vi "BLED1112-Rx Packet parser (EVENT-Attribute Client).vi"(5 "message package":u8[](array[numeric])=[128, 13, 4, 5, 0, 18, 0, 1, 8, 32, 32, 51, 48, 49, 54, 13, 10] format="%02x") -> (0 "message out":u8[](array[numeric])=[128, 13, 4, 5, 0, 18, 0, 1, 8, 32, 32, 51, 48, 49, 54, 13, 10] format="%02x", 1 "Packet OK":bool, 2 "Data Structure":T1={"Message Type (Response)"=128, "Payload length"=16, "Command Class (System)"=3, "Message ID"=0, "Connection handle"=0, "Attribute handle"=50697, "Attribute type"=109, "Attribute value (data)"=[234, 23, 0, 0, 6, 0, 100, 0, 0, 0, 255]} {"Attribute type" format="%02x" items=["read", "notify", "indicate", "read_by_type", "read_blob", "indicate_rsp_req"]; "Attribute value (data)" format="%02x"; "Attribute handle" format="%04x"; "Connection handle" format="%02x"; "Message ID" format="%02x"; "Message Type (Response)" format="%02x" items=["Command / Response"=0, "Event"=128]; "Command Class (System)" format="%02x" items=["System", "Persistent Store", "Attribute database", "Connection", "Attribute client", "Security Manager", "Generic Access Profile", "Hardware"]})   [LabVIEW 2015]
uses:
  Control-BLED Rx (EVENT-Attribute Client).ctl
  Lib_Bled112 toolkit/type_def/message_type.ctl
  Lib_Bled112 toolkit/type_def/message_class.ctl
panel:
  # "Rx Packet parser (EVENT-Attribute Client)"
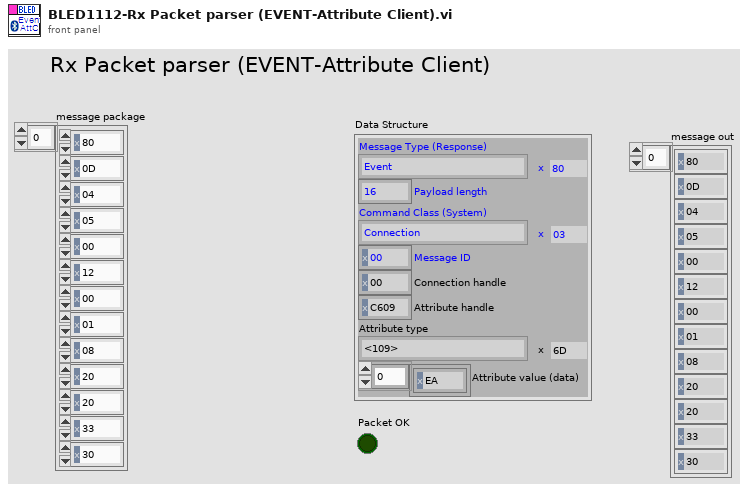
[diagram p1: front panel]
types:
  T1 = typedef "Control-BLED Rx (EVENT-Attribute Client).ctl" = cluster{"Message Type (Response)":T2, "Payload length":u8, "Command Class (System)":T3, "Message ID":u8, "Connection handle":u8, "Attribute handle":u16, "Attribute type":T3, "Attribute value (data)":u8[]}
  T2 = typedef "message_type.ctl" = u8
  T3 = typedef "message_class.ctl" = u8
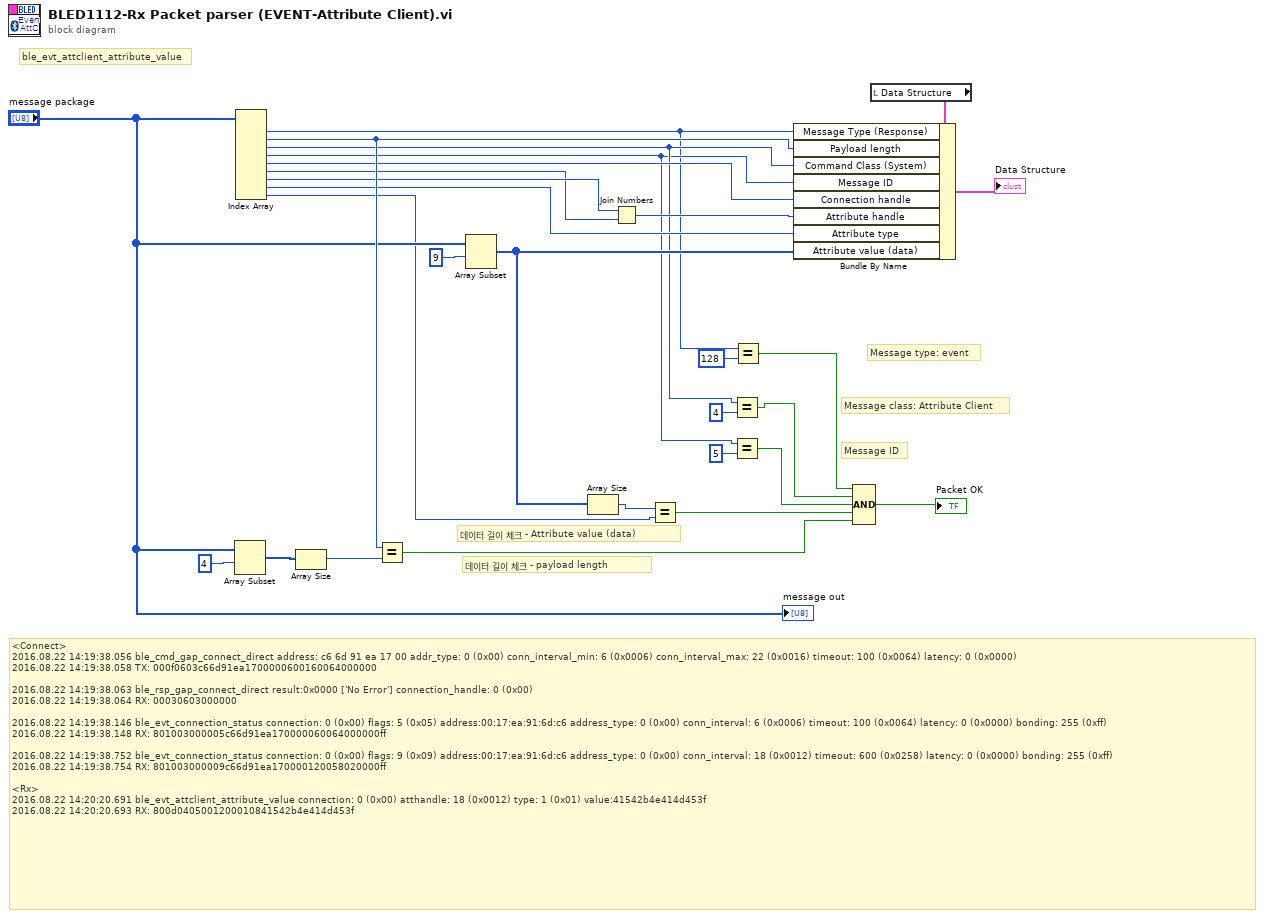
[diagram p0: block diagram]
diagram:
  # "Message type: event"
  # "Message ID"
  # "Message class: Attribute Client"
  # "데이터 길이 체크 - payload length"
  # "ble_evt_attclient_attribute_value"
  # "데이터 길이 체크 - Attribute value (data)"
  # "<Connect>\n2016.08.22 14:19:38.056 ble_cmd_gap_connect_direct address: c6 6d 91 ea 17 00 addr_type: 0 (0x00) conn_interval_min: 6 (0x0006) conn_interval_max: 22 (0x0016) timeout: 100 (0x0064) latency: 0 (0x0000)\n2016.08.22 14:19:38.058 TX: 000f0603c66d91ea1700000600160064000000\n\n2016.08.22 14:19:38.063 ble_rsp_gap_connect_direct result:0x0000 ['No Error'] connection_handle: 0 (0x00)\n2016.08.22 14:19:38.064 RX: 00030603000000\n\n2016.08.22 14:19:38.146 ble_evt_connection_status connection: 0 (0x00) flags: 5 (0x05) address:00:17:ea:91:6d:c6 address_type: 0 (0x00) conn_interval: 6 (0x0006) timeout: 100 (0x0064) latency: 0 (0x0000) bonding: 255 (0xff)\n2016.08.22 14:19:38.148 RX: 801003000005c66d91ea170000060064000000ff\n\n2016.08.22 14:19:38.752 ble_evt_connection_status connection: 0 (0x00) flags: 9 (0x09) address:00:17:ea:91:6d:c6 address_type: 0 (0x00) conn_interval: 18 (0x0012) timeout: 600 (0x0258) latency: 0 (0x0000) bonding: 255 (0xff)\n2016.08.22 14:19:38.754 RX: 801003000009c66d91ea170000120058020000ff\n\n<Rx>\n2016.08.22 14:20:20.691 ble_evt_attclient_attribute_value connection: 0 (0x00) atthandle: 18 (0x0012) type: 1 (0x01) value:41542b4e414d453f\n2016.08.22 14:20:20.693 RX: 800d0405001200010841542b4e414d453f"
  n1 = Array Subset(array="message package", index=4 ("인덱스")) -> (w16:u8[])  [unwired: 1 in]
  n2 = Index Array(array="message package") -> (element #1=w1:u8, element #2=w26:u8, element #3=w5:u8, element #4=w4:u8, element #5=w25:u8, element #6=w23:u8, element #7=w24:u8, element #8=w20:u8, element #9=w8:u8)  [unwired: 9 in]
  n3 = Array Size(array=w16) -> (size(s)=w15:i32)
  n4 = Equal?(x=w26, y=w15) -> (x = y?=w7:bool)
  n5 = Array Subset(array="message package", index=9 ("인덱스")) -> (w19:u8[])  [unwired: 1 in]
  n6 = Array Size(array=w19) -> (size(s)=w18:i32)
  n7 = Join Numbers(hi=w24, lo=w23) -> ((hi.lo)=w22:u16)
  n8 = Equal?(x=w18, y=w8) -> (x = y?=w6:bool)
  n9 = Equal?(x=w5, y=4 ("인덱스")) -> (x = y?=w10:bool)
  n10 = Equal?(x=w4, y=5 ("인덱스")) -> (x = y?=w11:bool)
  n11 = Equal?(x=w1, y=128 ("인덱스")) -> (x = y?=w2:bool)
  n12 = Compound Arithmetic op=AND ("복합 연산")(w2, w10, w11, w6, w7) -> (→"Packet OK":bool)
  n13 = local read "Data Structure"() -> (w28:T1)
  n14 = Bundle By Name(cluster=w28, "Message Type (Response)"=w1, "Payload length"=w26, "Command Class (System)"=w5, "Message ID"=w4, "Connection handle"=w25, "Attribute handle"=w22, "Attribute type"=w20, "Attribute value (data)"=w19) -> (→"Data Structure":T1)
  "message out" <- "message package"
